vi "PH_PILS.Action _OperationMode.vi"(0 "i ref in":refnum<vi>, 5 "error IO":errorcluster) -> (14 "i ref out":refnum<vi>, 19 "error out":errorcluster)   [LabVIEW 2014, in "PH_PILS.lvlib"]
doc: "This Vi calculates the operation mode."
uses:
  PH_PILS.lvlib
  PH_PILS.Operation Mode.ctl
  PH_Basics/PH_Common/PH_Common.lvlib
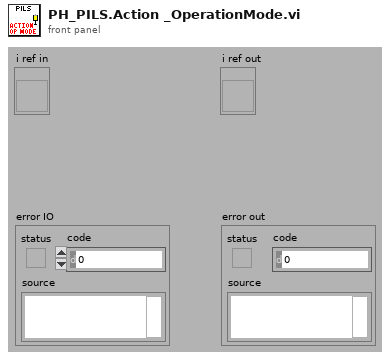
[diagram p1: front panel]
types:
  T1 = typedef "PH_PILS.lvlib/PH_PILS.i attribute.ctl" = cluster{"Boolean":cluster{"GUI Ref":refnum<vi>, "Status":i32}[], "GUI Refs Exp. Shutters":cluster{"1":refnum<vi>, "2":refnum<vi>, "3":refnum<vi>, "4":refnum<vi>}, "Tristate2Run GUI Refs":refnum<vi>[], "EO-Likes":cluster{"GUI Ref":refnum<vi>, "Status":i32}[], "Operation Mode":cluster{"Operation Mode":T2, "GUI":cluster{"Ref State":refnum<vi>, "Ref":refnum<vi>}, "Servicemode":cluster{"Tagname":string, "Status":i32}, "Labormode":cluster{"Tagname":string, "Status":i32}, "Searchmode":cluster{"Tagname":string, "Status":i32}, "Shotmode":cluster{"Tagname":string, "Status":i32}}, "Submode":cluster{"Submode":T3, "GUI":cluster{"Ref State":refnum<vi>, "Ref":refnum<vi>}, "Submode":cluster{"Tagname":string, "Status":i32}}, "Experiment":cluster{"Experiment":enum16{"unknown", "intern", "4 (Z6)", "3", "2", "1"}, "GUI":cluster{"Ref State":refnum<vi>, "Ref":refnum<vi>}, "intern":cluster{"Tagname":string, "Status":i32}, "Exp 4":cluster{"Tagname":string, "Status":i32}, "Exp 3":cluster{"Tagname":string, "Status":i32}, "Exp 2":cluster{"Tagname":string, "Status":i32}, "Exp 1":cluster{"Tagname":string, "Status":i32}}, "TristateNormal":cluster{"GUI Ref":refnum<vi>, "Status":i32}[], "Door Tags":cluster{"GUI Ref":refnum<vi>, "Status":i32}[], "GUIlessTags":cluster{"Name":string, "Status":i32}[], "Beamline GUI Refs":refnum<vi>[], "Special Boolean":cluster{"GUI Ref":refnum<vi>, "Status":i32}[], "Laserpower":cluster{"GUI Ref":refnum<vi>, "Status":i32}[], "Shutter":cluster{"GUI Ref":refnum<vi>, "Status":i32}[], "Tristate EO Like":cluster{"GUI Ref":refnum<vi>, "Status":i32}[], "PP":cluster{"GUI Ref":refnum<vi>, "Status":i32, "Head Ref":refnum<vi>, "Slider Ref":refnum<vi>}[], "Switch Knobs":cluster{"GUI Ref":refnum<vi>, "Status":i32}[], "Latch Knob GUI Refs":refnum<vi>[], "FailureCounter":i32, "Enabled Status":cluster{"Laser":i32, "PreAmp":i32, "MainAmp":i32}, "Mercury":refnum<vi>, "Instance Rods":string, "Logfile":path, "Beckhoff-Instance Internal":string, "Beckhoff-Instance External":string, "Enabling Rights":cluster{"Name":string, "Password":string, "PA?":bool, "MA?":bool, "Exp?":bool}[]}
  T2 = typedef "PH_PILS.lvlib/PH_PILS.Operation Mode.ctl" = enum16{"unknown", "Service", "Labor", "Search", "Shot"}
  T3 = typedef "PH_PILS.lvlib/PH_PILS.Submode.ctl" = enum16{"unknown", "HV-Normal", "HV-Test"}
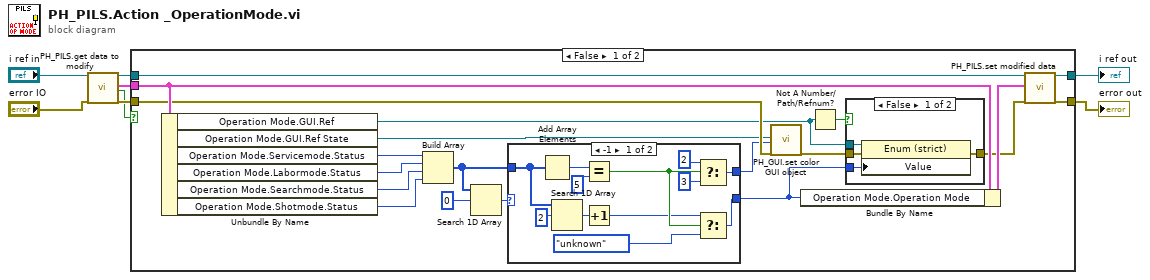
[diagram p0: block diagram]
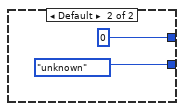
[diagram p2: hidden frame]
diagram:
  n1 = call "PH_PILS.get data to modify.vi"("i ref in"="i ref in", "error in (no error)"="error IO") -> ("i ref out"=w7:refnum<vi>, "i attribute"=w5:T1, "timed out"=w6:bool, "error out"=w8:errorcluster)  [unwired: 14 in]
  n2 = case shown="False" w6 {
    tunnel: [w28 w48] -> w3
    tunnel: w8 -> [w19 w48]
    tunnel: [w27 w49] -> w4
    tunnel: w7 -> [w26 w49]
    tunnel: w5 -> [w21 _]
    frame False {
      n3 = Unbundle By Name(w21) -> ("Operation Mode.GUI.Ref"=w14:refnum<vi>, "Operation Mode.GUI.Ref State"=w15:refnum<vi>, "Operation Mode.Servicemode.Status"=w25:i32, "Operation Mode.Labormode.Status"=w24:i32, "Operation Mode.Searchmode.Status"=w23:i32, "Operation Mode.Shotmode.Status"=w22:i32)
      n4 = Build Array(w25, w24, w23, w22) -> (w9:i32[])
      n5 = Search 1D Array(1D array=w9, element=0) -> (index of element=w12:i32)  [unwired: 1 in]
      n6 = case shown="-1" w12 {
        tunnel: [w33 PH_PILS.Operation_Mode."unknown" ("Operation Mode.Operation Mode")] -> w11
        tunnel: [w37 0 ("State")] -> w10
        tunnel: w9 -> [w32 _]
        frame -1 {
          n7 = Add Array Elements(numeric array=w32) -> (sum=w40:i32)
          n8 = Search 1D Array(1D array=w32, element=2) -> (index of element=w31:i32)  [unwired: 1 in]
          n9 = Equal?(x=w40, y=5) -> (x = y?=w35:bool)
          n10 = Increment(x=w31) -> (x+1=w29:i32)
          n11 = Select(t=2 ("State"), s=w35, f=3) -> (s? t:f=w37:i32)
          n12 = Select(t=w29, s=w35, f=PH_PILS.Operation_Mode."unknown" ("Operation Mode.Operation Mode")) -> (s? t:f=w33:i32)
        }
        frame Default {
        }
      }
      n13 = call "PH_GUI.set color GUI object.vi"("GUI object Ref"=w15, "State"=w10, "error in (no error)"=w19) -> ("error out"=w16:errorcluster)  [unwired: 16 in]
      n14 = Bundle By Name(cluster=w21, "Operation Mode.Operation Mode"=w11) -> (w20:T1)
      n15 = Not A Number/Path/Refnum?(number/path/refnum=w14) -> (NaN/Path/Refnum?=w17:bool)
      n16 = case shown="False" w17 {
        tunnel: w16 -> [w46 w47]
        tunnel: [w45 w47] -> w18
        tunnel: w14 -> [w44 _]
        tunnel: w11 -> [w43 _]
        frame False {
          n17 = property class="Enum (strict)"(reference=w44, error in=w46, "Value"=w43) -> (error out=w45:errorcluster)  [unwired: 1 out]
        }
        frame True {
        }
      }
      n18 = call "PH_PILS.set modified data.vi"("i ref in"=w26, "i attribute"=w20, "error in (no error)"=w18) -> ("i ref out"=w27:refnum<vi>, "error out"=w28:errorcluster)  [unwired: 15 in]
    }
    frame True {
    }
  }
  "error out" <- w3
  "i ref out" <- w4
